vi "GUI main 2.vi"() -> ()   [LabVIEW 2020]
uses:
  General PJVS driver/Type definitions/PJVS Type.ctl
  PJVS drivers/acsvcontrol-driver/build/ACSVcontrol-driver_0.2.0.0.llb/Debug status.ctl
  PJVS drivers/acsvcontrol-driver/build/ACSVcontrol-driver_0.2.0.0.llb/ACSVcontrol-driver.lvlib
  PJVS drivers/acsvcontrol-driver/build/ACSVcontrol-driver_0.2.0.0.llb/Timeouts.ctl
  General PJVS driver/Type definitions/PJVS Setup.ctl
panel:
  in  "PJVS setup":T1={"PJVS type"=enum."AC-supraVOLTcontrol", "Status Refnum"=refnum, "Abort Refnum"=refnum, "AC-supraVOLTcontrol"={"IP address:port (0.0.0.0:0000)"="0.0.0.0:0000", "Debug mode"=enum."No change", "Timeouts"={"TCP Read & Write (ms)"=7000, "Sensors readout"=5000, "PJVS setup"=10000, "Nullmeter readout"=5000, "Multiplexer setup"=3000, "57XX setup"=15000, "Generator setup"=5000, "Synthesizer setup"=3000, "Sampler readout"=10000}}, "NPL bias source"={"Server name"="CZC", "Bias setup file"=path ""}}
  in  "quit":bool
  in  "show pjvs setup":bool
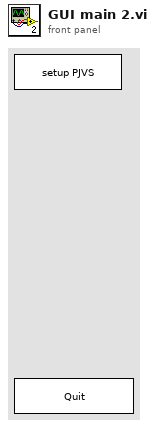
[diagram p1: front panel]
types:
  T1 = typedef "PJVS Setup.ctl" = cluster{"PJVS type":T2, "Status Refnum":refnum<vi>, "Abort Refnum":refnum<vi>, "AC-supraVOLTcontrol":cluster{"IP address:port (0.0.0.0:0000)":string, "Debug mode":T3, "Timeouts":T4}, "NPL bias source":cluster{"Server name":string, "Bias setup file":path}}
  T2 = typedef "PJVS Type.ctl" = enum16{"AC-supraVOLTcontrol", "NPL bias source"}
  T3 = typedef "ACSVcontrol-driver.lvlib/Debug status.ctl" = enum16{"No change", "Off", "On"}
  T4 = typedef "ACSVcontrol-driver.lvlib/Timeouts.ctl" = cluster{"TCP Read & Write (ms)":i32, "Sensors readout":i32, "PJVS setup":i32, "Nullmeter readout":i32, "Multiplexer setup":i32, "57XX setup":i32, "Generator setup":i32, "Synthesizer setup":i32, "Sampler readout":i32}
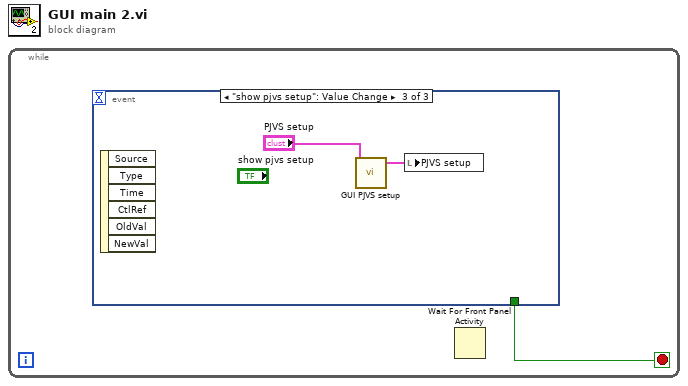
[diagram p0: block diagram]
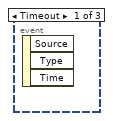
[diagram p2: hidden frame]
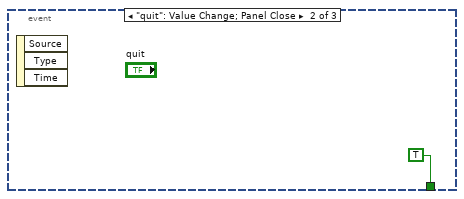
[diagram p3: hidden frame]
diagram:
  n1 = while {
    stop <- w1 stop-if-true
    n2 = event shown="[2] \"show pjvs setup\": Value Change" {
      selector: _ -> [_ _ _]
      dyn-events: _ -> [_ _ _]
      timeout: _ -> [_ _ _]
      tunnel: [_ TRUE _] -> w1
      event Timeout {
        n3 = event-data() -> ()  [unwired: 1 in, 3 out]
      }
      event "quit": Value Change; Panel Close {
        n4 = event-data() -> ()  [unwired: 1 in, 3 out]
      }
      event "show pjvs setup": Value Change {
        n5 = event-data() -> ()  [unwired: 1 in, 6 out]
        n6 = call "GUI PJVS setup.vi"("PJVS setup"="PJVS setup") -> ("PJVS setup out"=w3:T1)  [unwired: 10 in]
        n7 = local write "PJVS setup"(w3) -> ()
      }
    }
    n8 = Wait For Front Panel Activity() -> ()  [unwired: 3 in, 1 out]
  }
